vi "Add Message Response.vi"(8 "Error In":errorcluster, 11 "Message Refnum In":T1 format="%.0x") -> (0 "Error Out":errorcluster, 2 "Response Section Ptr":T1=18446744073709551615 format="%.0x", 3 "Message Refnum Out":T1 format="%.0x")   [LabVIEW 2020, in "Instrument Addon Scripting API.lvlib"]
uses:
  Instrument Addon Scripting API.lvlib
  <vilib>/NI VeriStand/Custom Device API/Custom Device Item Ref.ctl
  Shared Directory/Constants.vi
  Shared Directory/Instrument Addon Shared.lvlib
  <vilib>/NI VeriStand/Custom Device API/Custom Device API.lvlib
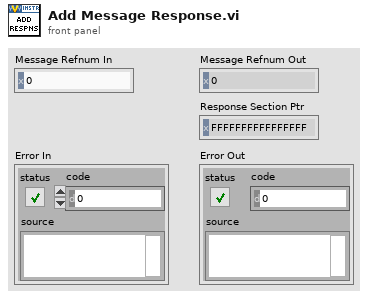
[diagram p1: front panel]
types:
  T1 = typedef "Custom Device API.lvlib/Custom Device Item Ref.ctl" = u64
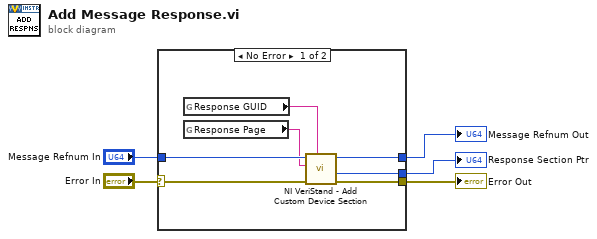
[diagram p0: block diagram]
diagram:
  n1 = case shown="No Error" "Error In" {
    selector: "Error In" -> [w7 w13]
    tunnel: [w12 w14] -> w2
    tunnel: [w11 w13] -> w1
    tunnel: "Message Refnum In" -> [w10 w14]
    tunnel: [w6 _] -> w3
    frame No Error {
      n2 = global read "Constants.vi" "Response GUID"() -> (w9:string)
      n3 = global read "Constants.vi" "Response Page"() -> (w8:string)
      n4 = call <vilib>:"NI VeriStand - Add Custom Device Section.vi"("GUID (Default Section)"=w9, "error in (no error)"=w7, "Section Name"=w8, "Parent Ref in"=w10) -> ("error out"=w11:errorcluster, "Section Ptr"=w6:T1, "Parent Ref out"=w12:T1)  [unwired: 4 in, 1 out]
    }
    frame Error {
    }
  }
  "Message Refnum Out" <- w2
  "Error Out" <- w1
  "Response Section Ptr" <- w3
